vi "test_client_builder.vi"() -> ()   [LabVIEW 2020, in "reqwest_tests.lvlib"]
uses:
  reqwest_tests.lvlib
  <vilib>/addons/_JKI Toolkits/Caraya/classes/Assert/Assert.lvclass
  <vilib>/addons/_JKI Toolkits/Caraya/classes/Test/Test.lvclass
  ClientBuilder/ClientBuilder.lvclass
  Client/Client.lvclass
panel:
  in  "error in (no error)":errorcluster
  out "error out":errorcluster
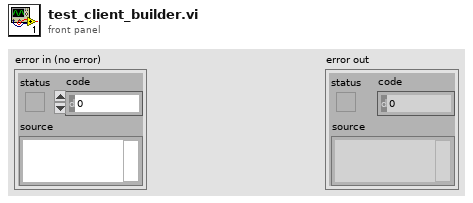
[diagram p1: front panel]
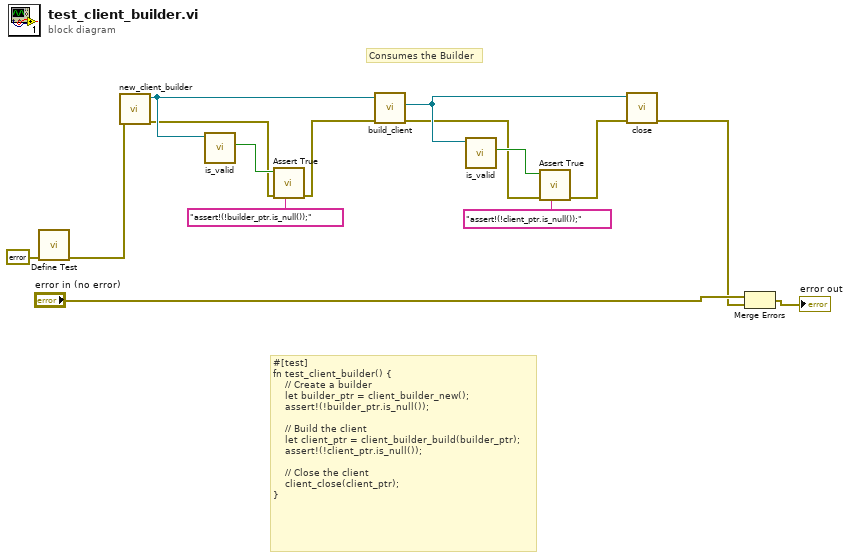
[diagram p0: block diagram]
diagram:
  # "Consumes the Builder"
  # "#[test]\nfn test_client_builder() {\n    // Create a builder\n    let builder_ptr = client_builder_new();\n    assert!(!builder_ptr.is_null());\n\n    // Build the client\n    let client_ptr = client_builder_build(builder_ptr);\n    assert!(!client_ptr.is_null());\n\n    // Close the client\n    client_close(client_ptr);\n}"
  n1 = call <vilib>:"Define Test.vi"("error in (no error)"=errorcluster {"status"=FALSE, "code"=0, "source"=""}) -> ("error out"=w5:errorcluster)  [unwired: 9 in, 1 out]
  n2 = call "new_client_builder.vi"("error in (no error)"=w5) -> ("error out"=w4:errorcluster, "Client out"=w10:refnum<class "ClientBuilder.lvclass">)  [unwired: 9 in]
  n3 = call "is_valid.vi"("Client in"=w10) -> ("valid-ref?"=w12:bool)  [unwired: 10 in]
  n4 = call <vilib>:"Assert True.vi"("Label"="assert!(!builder_ptr.is_null());", "error in (no error)"=w4, "True?"=w12) -> ("error out"=w3:errorcluster)  [unwired: 7 in, 1 out]
  n5 = call "build_client.vi"("error in (no error)"=w3, "ClientBuilder in"=w10) -> ("error out"=w2:errorcluster, "Client out"=w7:refnum<class "Client.lvclass">)  [unwired: 8 in]
  n6 = call "is_valid.vi"("Client in"=w7) -> ("valid-ref?"=w9:bool)  [unwired: 10 in]
  n7 = call <vilib>:"Assert True.vi"("Label"="assert!(!client_ptr.is_null());", "error in (no error)"=w2, "True?"=w9) -> ("error out"=w1:errorcluster)  [unwired: 7 in, 1 out]
  n8 = call "close.vi"("error in (no error)"=w1, "Client in"=w7) -> ("error out"=w6:errorcluster)  [unwired: 9 in]
  n9 = Merge Errors("error in (no error)", w6) -> (→"error out":errorcluster)
